vi "mxwScript_API_XMLMakeTemplateRefText.vi"(9 "referencePosition":T3, 10 "terminalData":T2, 11 "templateRefType":T1) -> (3 "templateRefText":string)   [LabVIEW 2017]
uses:
  codeGenAPISupport.llb/cgAPI_mxwScript_DrpTmplt_ReferencePosition.ctl
  codeGenAPISupport.llb/cgAPI_mxwScript_DrpTmplt_TerminalData.ctl
  codeGenAPISupport.llb/cgAPI_mxwScript_DrpTmplt_TemplateRefType.ctl
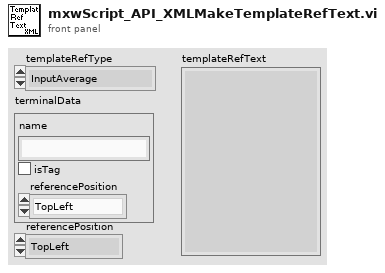
[diagram p1: front panel]
types:
  T1 = typedef "cgAPI_mxwScript_DrpTmplt_TemplateRefType.ctl" = enum16{"InputAverage", "Absolute", "Terminal"}
  T2 = typedef "cgAPI_mxwScript_DrpTmplt_TerminalData.ctl" = cluster{"name":string, "termIsTag":bool, "referencePosition":T3}
  T3 = typedef "cgAPI_mxwScript_DrpTmplt_ReferencePosition.ctl" = enum16{"TopLeft", "Top", "TopRight", "Left", "Middle", "Right", "BottomLeft", "Bottom", "BottomRight"}
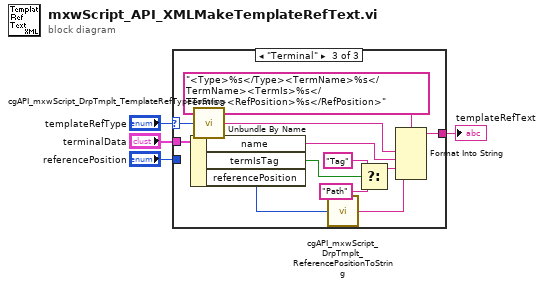
[diagram p0: block diagram]
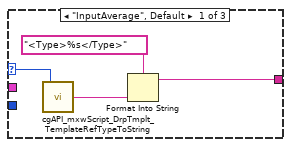
[diagram p2: hidden frame]
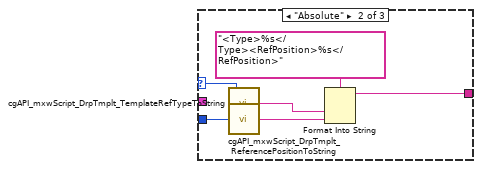
[diagram p3: hidden frame]
diagram:
  n1 = case shown="\"Terminal\"" "templateRefType" {
    selector: "templateRefType" -> [w6 w10 w18]
    tunnel: "terminalData" -> [_ _ w20]
    tunnel: "referencePosition" -> [_ w12 _]
    tunnel: [w7 w13 w21] -> w3
    frame "InputAverage", Default {
      n2 = call "cgAPI_mxwScript_DrpTmplt_TemplateRefTypeToString.vi"("templateRefType"=w6) -> ("string"=w5:string)  [unwired: 4 out]
      n3 = Format Into String(format string="<Type>%s</Type>", w5) -> (resulting string=w7:string)  [unwired: 2 in, 1 out]
    }
    frame "Absolute" {
      n4 = call "cgAPI_mxwScript_DrpTmplt_TemplateRefTypeToString.vi"("templateRefType"=w10) -> ("string"=w9:string)  [unwired: 4 out]
      n5 = call "cgAPI_mxwScript_DrpTmplt_ReferencePositionToString.vi"("referencePosition"=w12) -> ("string"=w11:string)  [unwired: 4 out]
      n6 = Format Into String(format string="<Type>%s</Type><RefPosition>%s</RefPosition>", w9, w11) -> (resulting string=w13:string)  [unwired: 2 in, 1 out]
    }
    frame "Terminal" {
      n7 = Unbundle By Name(w20) -> ("name"=w25:string, "termIsTag"=w24:bool, "referencePosition"=w15:T3)
      n8 = call "cgAPI_mxwScript_DrpTmplt_TemplateRefTypeToString.vi"("templateRefType"=w18) -> ("string"=w17:string)  [unwired: 4 out]
      n9 = call "cgAPI_mxwScript_DrpTmplt_ReferencePositionToString.vi"("referencePosition"=w15) -> ("string"=w16:string)  [unwired: 4 out]
      n10 = Select(t="Tag", s=w24, f="Path") -> (s? t:f=w19:string)
      n11 = Format Into String(format string="<Type>%s</Type><TermName>%s</TermName><TermIs>%s</TermIs><RefPosition>%s</RefPosition>", w17, w25, w19, w16) -> (resulting string=w21:string)  [unwired: 2 in, 1 out]
    }
  }
  "templateRefText" <- w3
